vi "1xKETTLE_Int.vi"() -> ()   [LabVIEW 2015]
uses:
  <vilib>/Platform/TimedLoop/XDataNode/XDataNode.xnode
  <vilib>/Platform/TimedLoop/XDataNode/nitl_modes.ctl
  <vilib>/Platform/TimedLoop/XDataNode/XDNodeRunTimeDep.lvlib
  <vilib>/Platform/TimedLoop/XDataNode/wakeup.ctl
  <vilib>/Platform/TimedLoop/XDataNode/timing_clust.ctl
  <vilib>/rvi/DataTransferAndStorage/Container/XNode/niFpgaContainer.xnode
  <vilib>/eio/EIONode/EIONode.xnode
  <vilib>/rvi/eio/common/nirviEmuTemplateMethod_errors.vi
  <vilib>/rvi/Memory/Memory_Emulation/nirvimemoryEmulation.vi
  <vilib>/rvi/Memory/Memory_Emulation/nirvimemoryFastEmulation.vi
  <vilib>/rvi/interface/RandomDataEmulation/nirviRandomDataFpgaReadWriteTemplate.vi
  <vilib>/rvi/FIFO/Fifo_Resource/nirvififoEmulationWrite.vi
  <vilib>/rvi/FIFO/Fifo_Resource/nirvififoEmulationRead.vi
panel:
  in  "1/2":bool
  in  "Scale":i8
  in  "Levels":u8
  in  "Delay?":bool
  in  "1/Attack":fxp<+,16,0>
  in  "1/Decay":fxp<+,16,0>
  in  "Sustain":fxp<+,16,0>
  in  "S/R":fxp<+,16,0>
  in  "Amount":fxp<+,8,0>
  in  "Gate":bool
  in  "LFO":fxp<+/-,8,8>
  out "VCA Out":i16
  in  "Init?":bool
  out "From Host?":bool
  out "To Host?":bool
  in  "Start":bool
  out "Recording":bool
  in  "Clear?":bool
  out "Flag":bool
  in  "Transfer":bool
  in  "M":fxp<+,32,32>
  in  "Trigger":bool
  # "VCO"
  # "EL KETTLE 2 NO ESTA CONSEGUIDO AUN!!!  =("
  # "VCA"
  # "Rep"
  # "Interf"
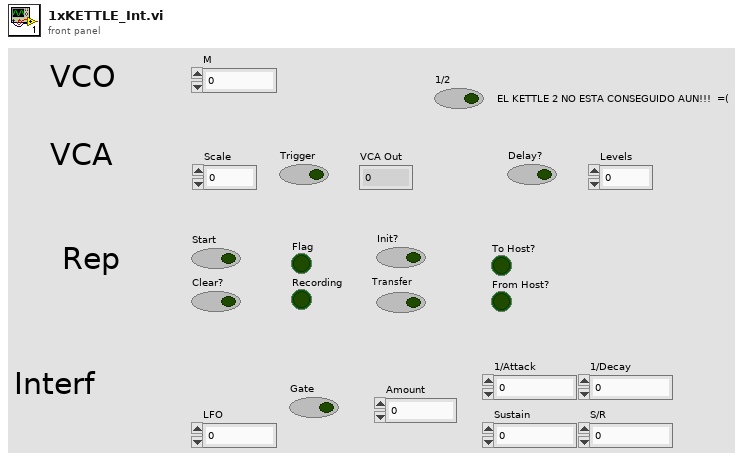
[diagram p1: front panel]
types:
  T1 = typedef "XDNodeRunTimeDep.lvlib/timing_clust.ctl" = cluster{"Expected End [f-1]":u64, "Actual End [f-1]":u64, "Finished Late? [f-1]":bool, "Expected End [i-1]":u64, "Actual End [i-1]":u64, "Finished Late? [i-1]":bool, "Expected Start [i]":u64, "Actual Start [i]":u64, "Expected Start [f]":u64, "Actual Start [f]":u64, "Source Name":string, "Structure Name":string, "Period":i64, "Deadline":i64, "Offset":i64, "Start":i64, "Priority":i32, "Timeout":i32, "Mode":T2, "Wakeup Reason":T3, "Error":errorcluster, "Source Type":string, "Secondary Source Type":string, "Global End Time":u64, "Global Start Time":u64, "Frame Duration":u64, "Iteration Duration":u64, "Assigned CPU":i32, "I/O Scan Engine Mode":u32}
  T2 = typedef "XDNodeRunTimeDep.lvlib/nitl_modes.ctl" = enum32{"No Change", "Process missed periods, maintain original phase", "Discard missed periods, maintain original phase", "Process missed periods, ignore original phase", "Discard missed periods, ignore original phase"}
  T3 = typedef "XDNodeRunTimeDep.lvlib/wakeup.ctl" = enum32{"Normal", "Aborted", "Asynchronous wakeup", "Timing source error", "Timed loop error", "Timeout"}
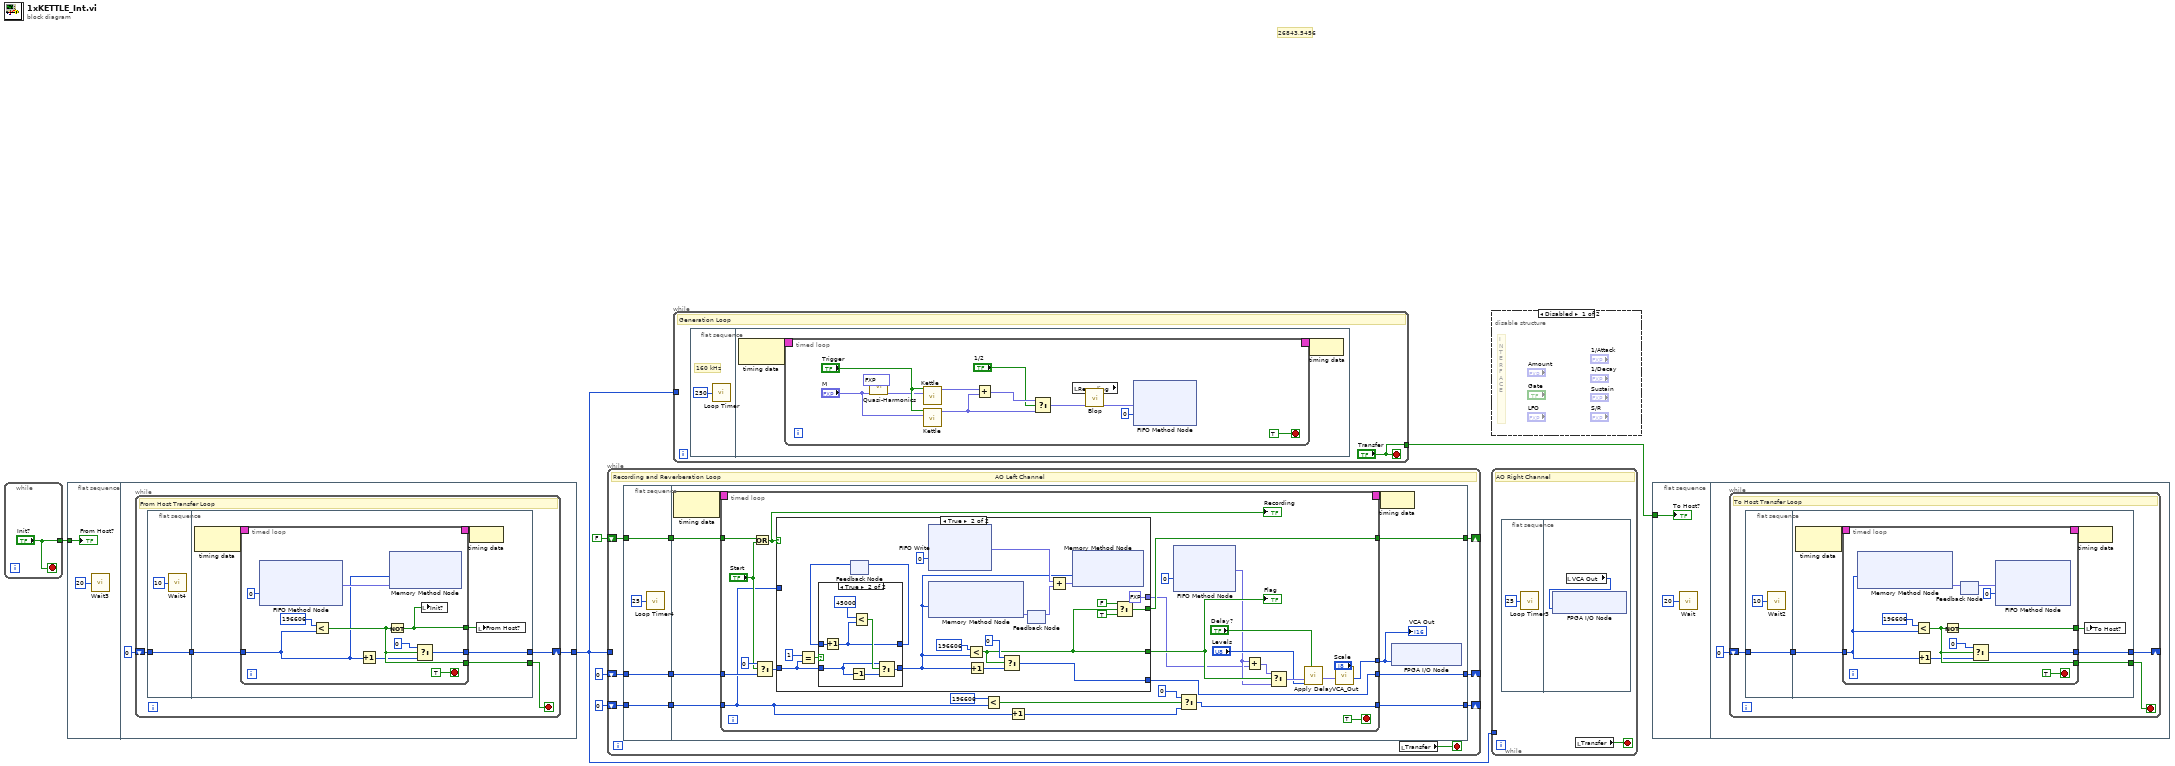
[diagram p0: block diagram]
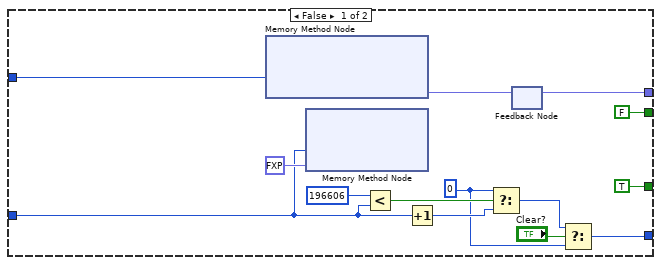
[diagram p3: hidden frame]
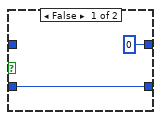
[diagram p4: hidden frame]
diagram:
  # "26843,5456"
  n1 = while {
    tunnel: ["Init?"] -> w4
    stop <- "Init?" stop-if-true
  }
  n2 = flat-sequence {
    tunnel: w4 -> [w9]
    tunnel: [w10] -> w3
    frame #0 {
      n3 = call "Wait3"("Count(mSec)"=u8 20) -> ()  [unwired: 1 out]
      "From Host?" <- w9
    }
    frame #1 {
      n4 = while {
        shift-right: [w13] -> w10
        shift-left: u32 0 -> [w14]
        stop <- w12 stop-if-true
        # "From Host Transfer Loop"
        n5 = flat-sequence {
          tunnel: [w17] -> w15
          tunnel: w14 -> [w17]
          tunnel: w15 -> [w21]
          tunnel: [w20] -> w13
          tunnel: [w19] -> w12
          frame #0 {
            n6 = call "Wait4"("Count(uSec)"=u8 10) -> ()  [unwired: 1 out]
          }
          frame #1 {
            n7 = node-c288() -> (w23:T1)  [unwired: 1 in]
            n8 = timed-loop {
              timing: w23 -> [_]
              timing-out: [_] -> w22
              tunnel: w21 -> [w26]
              tunnel: [w29] -> w19
              tunnel: [w28] -> w20
              tunnel: [w24] -> w18
              stop <- TRUE stop-if-true
              n9 = xnode ("FIFO Method Node")("Timeout"=0) -> ("Element"=w33:fxp<+/-,8,8>)  [unwired: 1 in, 2 out]
              n10 = Less?(x=u32 196606, y=w26) -> (x < y?=w29:bool)
              n11 = Increment(x=w26) -> (x+1=w25:u32)
              n12 = Not(x=w29) -> (.not. x?=w24:bool)
              n13 = xnode ("Memory Method Node")("Address"=w26, "Data"=w33) -> ()  [unwired: 1 in, 1 out]
              n14 = Select(t=u32 0, s=w29, f=w25) -> (s? t:f=w28:u32)
              n15 = local write "Init?"(w24) -> ()
            }
            n16 = node-c288(w22) -> ()
            n17 = local write "From Host?"(w18) -> ()
          }
        }
      }
    }
  }
  n18 = while {
    shift-right: [w38] -> _
    shift-left: u32 0 ("Address") -> [w46]
    shift-right: [w43] -> _
    shift-left: FALSE ("t") -> [w44]
    tunnel: w3 -> [_]
    shift-right: [w39] -> _
    shift-left: u32 0 ("Address") -> [w40]
    stop <- w42 stop-if-true
    # "Recording and Reverberation Loop                                                                                                                                         AO Left Channel"
    n19 = flat-sequence {
      tunnel: [w50] -> w47
      tunnel: w46 -> [w50]
      tunnel: w44 -> [w49]
      tunnel: [w49] -> w45
      tunnel: [w48] -> w41
      tunnel: w40 -> [w48]
      tunnel: w47 -> [w60]
      tunnel: w45 -> [w59]
      tunnel: [w58] -> w43
      tunnel: w41 -> [w55]
      tunnel: [w54] -> w39
      tunnel: [w52] -> w38
      frame #0 {
        n20 = call "Loop Timer4"("Count(uSec)"=u8 25) -> ()  [unwired: 1 out]
      }
      frame #1 {
        n21 = node-c288() -> (w57:T1)  [unwired: 1 in]
        n22 = timed-loop {
          timing: w57 -> [_]
          timing-out: [_] -> w56
          tunnel: w60 -> [w71]
          tunnel: w59 -> [w69]
          tunnel: [w67] -> w58
          tunnel: w55 -> [w62]
          tunnel: [w75] -> w54
          tunnel: [w74] -> w53
          tunnel: [w65] -> w52
          stop <- TRUE stop-if-true
          n23 = Or(x=w69, y="Start") -> (x .or. y?=w68:bool)
          "Recording" <- w68
          n24 = Select(t=u32 0, s="Start", f=w71) -> (s? t:f=w72:u32)
          n25 = case shown="True" w68 {
            tunnel: [w100 w112] -> w65
            tunnel: w72 -> [w94 w105]
            tunnel: [FALSE ("t") w119] -> w67
            tunnel: [TRUE w108] -> w66
            tunnel: w62 -> [w92 _]
            tunnel: [w90 fxp<+/-,8,8> 0.0 ("Data")] -> w61
            frame False {
              w89 = u32 0 ("y")
              n26 = xnode ("Memory Method Node")("Address"=w92) -> ("Data"=w91:fxp<+/-,8,8>)  [unwired: 1 in, 1 out]
              n27 = xnode ("Memory Method Node")("Address"=w94, "Data"=fxp<+/-,8,8> 0.0) -> ()  [unwired: 1 in, 1 out]
              n28 = Less?(x=u32 196606 ("y"), y=w94) -> (x < y?=w99:bool)
              n29 = Increment(x=w94) -> (x+1=w95:u32)
              n30 = Select(t=w89, s=w99, f=w95) -> (s? t:f=w97:u32)
              n31 = feedback #1() -> (w90:fxp<+/-,8,8>)  [unwired: 1 in]
              n32 = feedback-in #1(w91) -> ()
              n33 = Select(t=w97, s="Clear?", f=w89) -> (s? t:f=w100:u32)
            }
            frame True {
              n34 = Equal?(x=u32 1, y=w105) -> (x = y?=w106:bool)
              n35 = feedback #2() -> (w101:u32)  [unwired: 1 in]
              n36 = case shown="True" w106 {
                tunnel: w105 -> [w122 w124]
                tunnel: [w122 w128] -> w103
                tunnel: [u32 0 w123] -> w102
                tunnel: w101 -> [_ w129]
                frame False {
                }
                frame True {
                  n37 = Increment(x=w129) -> (x+1=w123:u32)
                  n38 = Decrement(x=w124) -> (x-1=w125:u32)
                  n39 = Less?(x=u32 45000 ("End"), y=w123) -> (x < y?=w126:bool)
                  n40 = Select(t=w124, s=w126, f=w125) -> (s? t:f=w128:u32)
                }
              }
              n41 = feedback-in #2(w102) -> ()
              n42 = xnode ("FIFO Write")("Timeout"=0) -> ("Element"=w115:fxp<+/-,8,8>)  [unwired: 1 in, 2 out]
              n43 = xnode ("Memory Method Node")("Address"=w103) -> ("Data"=w113:fxp<+/-,8,8>)  [unwired: 1 in, 1 out]
              n44 = Less?(x=u32 196606 ("y"), y=w103) -> (x < y?=w108:bool)
              n45 = Increment(x=w103) -> (x+1=w116:u32)
              n46 = Select(t=u32 0, s=w108, f=w116) -> (s? t:f=w112:u32)
              n47 = feedback-in #3(w113) -> ()
              n48 = feedback #3() -> (w109:fxp<+/-,8,8>)  [unwired: 1 in]
              n49 = Add(x=w115, y=w109) -> (x+y=w114:fxp<+/-,8,8>)
              n50 = xnode ("Memory Method Node")("Address"=w103, "Data"=w114) -> ()  [unwired: 1 in, 1 out]
              n51 = Select(t=FALSE, s=w108, f=TRUE) -> (s? t:f=w119:bool)
            }
          }
          "Flag" <- w66
          n52 = Less?(x=u32 196606, y=w62) -> (x < y?=w78:bool)
          n53 = Increment(x=w62) -> (x+1=w80:u32)
          n54 = xnode ("FIFO Method Node")("Timeout"=0) -> ("Element"=w63:fxp<+/-,8,8>)  [unwired: 1 in, 2 out]
          n55 = Select(t=u32 0, s=w78, f=w80) -> (s? t:f=w75:u32)
          n56 = Add(x=w63, y=w61) -> (x+y=w64:fxp<+/-,8,8>)
          n57 = Select(t=w64, s=w66, f=w63) -> (s? t:f=w84:fxp<+/-,8,8>)
          n58 = call "Apply Delay.vi"("Delay?"="Delay?", "Levels"="Levels", "Element in"=w84) -> ("Element out"=w85:fxp<+/-,8,8>)  [unwired: 8 in]
          n59 = call "VCA_Out.vi"("Scale"="Scale", "Sample In"=w85) -> ("Sample Out"=w74:i16)  [unwired: 9 in]
        }
        "VCA Out" <- w53
        n60 = node-c288(w56) -> ()
        n61 = xnode "FPGA I/O Node"("AudioOut/Left"=w53) -> ()  [unwired: 1 in, 1 out]
      }
    }
    n62 = local read "Transfer"() -> (w42:bool)
  }
  n63 = while {
    tunnel: w3 -> [_]
    tunnel: ["Transfer"] -> w1
    stop <- "Transfer" stop-if-true
    # "Generation Loop"
    n64 = flat-sequence {
      frame #0 {
        # "160 kHz"
        n65 = call "Loop Timer"("Count(Ticks)"=u8 250) -> ()  [unwired: 1 out]
      }
      frame #1 {
        n66 = node-c288() -> (w137:T1)  [unwired: 1 in]
        n67 = timed-loop {
          timing: w137 -> [_]
          timing-out: [_] -> w136
          stop <- TRUE stop-if-true
          n68 = call "Quasi-Harmonics.vi"("Relative Freq"=fxp<+,8,3> 2.03125 ("relative f"), "1st partial"="M") -> ("Result Partial"=w145:fxp<+,32,32>)  [unwired: 9 in]
          n69 = call "Kettle.vi"("M"=w145, "Trigger"="Trigger") -> ("Kettle 1 Out"=w142:fxp<+/-,8,8>)  [unwired: 9 in]
          n70 = call "Kettle.vi"("M"="M", "Trigger"="Trigger") -> ("Kettle 1 Out"=w141:fxp<+/-,8,8>)  [unwired: 9 in]
          n71 = Add(x=w142, y=w141) -> (x+y=w140:fxp<+/-,8,8>)
          n72 = Select(t=w140, s="1/2", f=w141) -> (s? t:f=w138:fxp<+/-,8,8>)
          n73 = local read "Recording"() -> (w147:bool)
          n74 = call "Blop.vi"("Rec"=w147, "Sample In"=w138) -> ("Sample Out"=w148:fxp<+/-,8,8>)  [unwired: 9 in]
          n75 = xnode ("FIFO Method Node")("Element"=w148, "Timeout"=0) -> ()  [unwired: 1 in, 2 out]
        }
        n76 = node-c288(w136) -> ()
      }
    }
  }
  n77 = disable-structure shown="Disabled" {
    frame Disabled {
      # "I\nN\nT\nE\nR\nF\nA\nC\nE"
    }
    frame Enabled {
    }
  }
  n78 = while {
    tunnel: w3 -> [_]
    stop <- w155 stop-if-true
    # "AO Right Channel"
    n79 = flat-sequence {
      frame #0 {
        n80 = call "Loop Timer3"("Count(uSec)"=u8 25) -> ()  [unwired: 1 out]
      }
      frame #1 {
        n81 = local read "VCA Out"() -> (w157:i16)
        n82 = xnode "FPGA I/O Node"("AudioOut/Right"=w157) -> ()  [unwired: 1 in, 1 out]
      }
    }
    n83 = local read "Transfer"() -> (w155:bool)
  }
  n84 = flat-sequence {
    tunnel: w1 -> [w159]
    frame #0 {
      n85 = call "Wait"("Count(mSec)"=u8 20) -> ()  [unwired: 1 out]
      "To Host?" <- w159
    }
    frame #1 {
      n86 = while {
        shift-right: [w162] -> _
        shift-left: u32 0 -> [w163]
        stop <- w161 stop-if-true
        # "To Host Transfer Loop"
        n87 = flat-sequence {
          tunnel: [w166] -> w164
          tunnel: w163 -> [w166]
          tunnel: w164 -> [w170]
          tunnel: [w169] -> w162
          tunnel: [w168] -> w161
          frame #0 {
            n88 = call "Wait2"("Count(uSec)"=u8 10) -> ()  [unwired: 1 out]
          }
          frame #1 {
            n89 = node-c288() -> (w172:T1)  [unwired: 1 in]
            n90 = timed-loop {
              timing: w172 -> [_]
              timing-out: [_] -> w171
              tunnel: w170 -> [w176]
              tunnel: [w181] -> w168
              tunnel: [w180] -> w169
              tunnel: [w173] -> w167
              stop <- TRUE stop-if-true
              n91 = xnode ("Memory Method Node")("Address"=w176) -> ("Data"=w175:fxp<+/-,8,8>)  [unwired: 1 in, 1 out]
              n92 = Less?(x=u32 196606, y=w176) -> (x < y?=w181:bool)
              n93 = Increment(x=w176) -> (x+1=w178:u32)
              n94 = Not(x=w181) -> (.not. x?=w173:bool)
              n95 = feedback-in #4(w175) -> ()
              n96 = feedback #4() -> (w174:fxp<+/-,8,8>)  [unwired: 1 in]
              n97 = Select(t=u32 0, s=w181, f=w178) -> (s? t:f=w180:u32)
              n98 = xnode ("FIFO Method Node")("Element"=w174, "Timeout"=0) -> ()  [unwired: 1 in, 2 out]
            }
            n99 = node-c288(w171) -> ()
            n100 = local write "To Host?"(w167) -> ()
          }
        }
      }
    }
  }
